vi "GetCustomDeviceTimingSourceVIs.vi"(8 "error in (no error)":errorcluster, 11 "custom device reference in":refnum<k24>) -> (0 "error out":errorcluster, 2 "timing source VIs":cluster{"Location":refnum<k24>, path}[](array[cluster]), 3 "custom device reference out":refnum<k24>)   [LabVIEW 2016, in "VeriStandTestUtilities.lvlib"]
uses:
  VeriStandTestUtilities.lvlib
  NationalInstruments.VeriStand.XMLReader
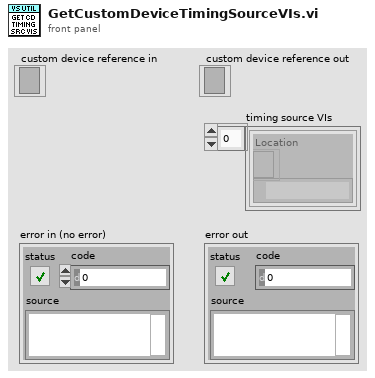
[diagram p1: front panel]
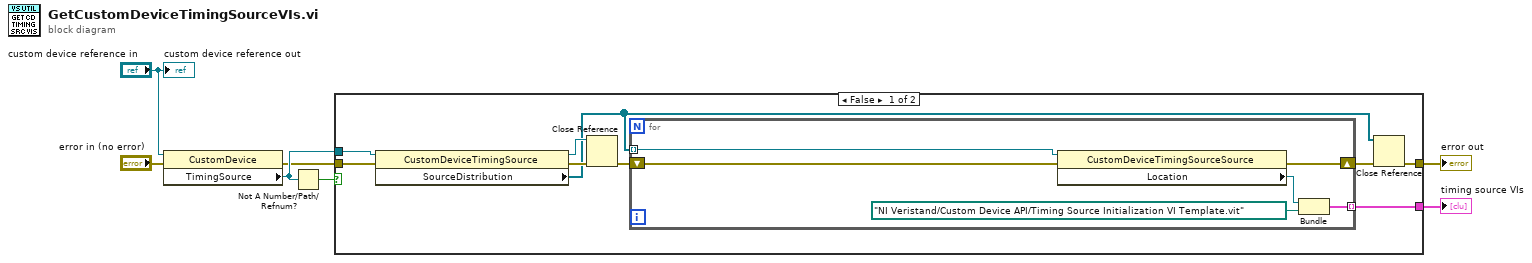
[diagram p0: block diagram]
diagram:
  n1 = property class="CustomDevice"(reference="custom device reference in", error in="error in (no error)") -> (error out=w2:errorcluster, "TimingSource"=w4:refnum<k24>)  [unwired: 1 out]
  n2 = Not A Number/Path/Refnum?(number/path/refnum=w4) -> (NaN/Path/Refnum?=w5:bool)
  n3 = case shown="False" w5 {
    tunnel: w4 -> [w16 _]
    tunnel: [w15 _] -> w7
    tunnel: w2 -> [w14 w23]
    tunnel: [w9 w23] -> w1
    frame False {
      n4 = property class="CustomDeviceTimingSource"(reference=w16, error in=w14) -> (reference out=w10:refnum<k24>, error out=w13:errorcluster, "SourceDistribution"=w8:refnum<k24>[])
      n5 = Close Reference(reference=w10, error in (no error)=w13) -> (error out=w11:errorcluster)
      n6 = for {
        tunnel: w8 -> [w22] mode=indexing
        tunnel: [w19] -> w15 mode=indexing
        shift-right: [w17] -> w12
        shift-left: w11 -> [w18]
        n7 = property class="CustomDeviceTimingSourceSource"(reference=w22, error in=w18) -> (error out=w17:errorcluster, "Location"=w21:refnum<k24>)  [unwired: 1 out]
        n8 = Bundle("Location"=w21, path "NI Veristand/Custom Device API/Timing Source Initialization VI Template.vit") -> (w19:cluster{"Location":refnum<k24>, path})  [unwired: 1 in]
      }
      n9 = Close Reference(reference=w8, error in (no error)=w12) -> (error out=w9:errorcluster)
    }
    frame True {
    }
  }
  "timing source VIs" <- w7
  "error out" <- w1
  "custom device reference out" <- "custom device reference in"
